vi "PRISM_RasterScan_BSC202.vi"() -> ()   [LabVIEW 2022 SP3]
uses:
  C:/Users/mnopl/Desktop/Software/mnOPSuite/PRISM/Thorlabs.MotionControl.Controls.dll
  Thorlabs.MotionControl.Controls.dll
  C:/Users/mnopl/Desktop/Software/mnOPSuite/PRISM/Thorlabs.MotionControl.Benchtop.StepperMotorCLI.dll
  Thorlabs.MotionControl.Benchtop.StepperMotorCLI.dll
  Control_PRISMRasterScan_ActivityLoop.ctl
  Control_PRISMRasterScan_ProtocolsLoop.ctl
  Control_LineScanCounterAE.ctl
  <vilib>/Analysis/baseanly.llb/Mean (DBL).vi
  C:/Users/mnopl/Desktop/Software/mnOPSuite/PRISM/Thorlabs.MotionControl.KCube.StepperMotorCLI.dll
  Thorlabs.MotionControl.KCube.StepperMotorCLI.dll
  <vilib>/Analysis/NI_AALBase.lvlib
panel:
  in  "Update origin":bool
  out "Protocol status":string="Ready for protocol!"
  in  "Protocols":T1(tab)
  in  "Target coordinate":T2={"X coord (mm)"=10.4027, "Y coord (mm)"=14.895, "Z coord (mm)"=19.058}
  in  "Move to target":bool
  out "Origin coordinate":T2={"X coord (mm)"=10.4027001953125, "Y coord (mm)"=14.895, "Z coord (mm)"=19.057761655908987}
  in  "Update target":bool
  in  "Move to origin":bool
  in  "Stored positions":T3(array[cluster])=[{"X coord (mm)"=10.4027, "Y coord (mm)"=14.895, "Z coord (mm)"=19.058}, {"X coord (mm)"=4.4859619140625, "Y coord (mm)"=8.22592529296875, "Z coord (mm)"=18.22813350697374}, {"X coord (mm)"=9.08337158203125, "Y coord (mm)"=16.38648681640625, "Z coord (mm)"=19.027052048324006}]
  in  "Stored position names":string[](array[string])=["SSO Center", "Gold", "Shane region"]
  in  "Move to\nstored position":bool[](array[boolean])=[FALSE, FALSE, FALSE]
  in  "Store target\nposition to":bool[](array[boolean])=[FALSE, FALSE, FALSE]
  in  "Do Linescan":bool
  in  "Linescan points\n(relative x,y, microns)":dbl[][](array[numeric])=[[1973.4850685095644, -1528.847563473508], [1962.5356538406427, -1517.3322023102946], [1951.5862391717208, -1505.8168411470815], [1940.636824502799, -1494.3014799838681], [1929.6874098338772, -1482.786118820655], [1918.7379951649555, -1471.2707576574417], [1907.7885804960335, -1459.7553964942285], [1896.8391658271119, -1448.2400353310152], [1885.88975115819, -1436.7246741678018], [1874.9403364892682, -1425.2093130045887], [1863.9909218203463, -1413.6939518413753], [1853.0415071514246, -1402.1785906781622], [1842.0920924825027, -1390.6632295149489], [1831.142677813581, -1379.1478683517357], [1820.193263144659, -1367.6325071885224], [1809.2438484757374, -1356.117146025309], [1798.2944338068155, -1344.6017848620959], [1787.3450191378938, -1333.0864236988825], [1776.395604468972, -1321.5710625356694], [1765.4461898000502, -1310.055701372456], [1754.4967751311283, -1298.540340209243], [1743.5473604622066, -1287.0249790460296], [1732.597945793285, -1275.5096178828162], [1721.648531124363, -1263.994256719603], [1710.699116455441, -1252.4788955563897], [1699.7497017865194, -1240.9635343931764], [1688.8002871175977, -1229.4481732299632], [1677.8508724486758, -1217.93281206675], [1666.901457779754, -1206.4174509035367], [1655.9520431108322, -1194.9020897403234], [1645.0026284419105, -1183.3867285771103], [1634.0532137729886, -1171.871367413897], [1623.1037991040669, -1160.3560062506835], [1612.154384435145, -1148.8406450874704], [1601.2049697662233, -1137.325283924257], [1590.2555550973013, -1125.809922761044], [1579.3061404283796, -1114.2945615978306], [1568.3567257594577, -1102.7792004346175], [1557.407311090536, -1091.263839271404], [1546.4578964216144, -1079.7484781081907], [1535.5084817526924, -1068.2331169449776], [1524.5590670837705, -1056.7177557817643], [1513.6096524148488, -1045.2023946185511], [1502.6602377459271, -1033.6870334553378], [1491.7108230770052, -1022.1716722921245], [1480.7614084080833, -1010.6563111289113], [1469.8119937391616, -999.140949965698], [1458.86257907024, -987.6255888024848], [1447.913164401318, -976.1102276392714], [1436.963749732396, -964.5948664760582], [1426.0143350634744, -953.079505312845], [1415.0649203945527, -941.5641441496317], [1404.1155057256308, -930.0487829864185], [1393.1660910567089, -918.5334218232052], [1382.2166763877872, -907.018060659992], [1371.2672617188655, -895.5026994967786], [1360.3178470499438, -883.9873383335654], [1349.3684323810219, -872.4719771703521], [1338.4190177121, -860.9566160071389], [1327.4696030431783, -849.4412548439257]]
  in  "Linescan Accumulations":i32=10 min=1
  out "Current point":i32
  in  "Halt linescan":bool
  out "Current\naccumulation":i32=10
  in  "Generate\n# points\n(cursors 1&2)":bool
  in  "# Points":i32=60 min=2 max=100
  out "X stepper reference":refnum<k24>
  out "Y stepper reference":refnum<k24>
  in  "BenchtopStepperControl Y":refnum<k24>(container)
  in  "BenchtopStepperControl X":refnum<k24>(container)
  in  "Save Image":bool
  in  "Path to save image":path=path "D:/Dropbox/Data/PRISM/2022.12.15 - SSO film undopded - test linescans/SSO(Overall)@(14.25microns,Mono,45degrees)_phase.txt"
  in  "Move to cursor 1":bool
  in  "Auto-level phase":bool
  in  "Acquire":bool=TRUE
  in  "Settle Time Y":u32=500
  in  "2nd sideband factor":dbl=1.0
  in  "Settle Time X":u32=50
  in  "Py":dbl=1.385597069551572 format="%_3f"
  in  "Px":dbl=-9.353762914113396 format="%_3f"
  in  "1st sideband offset":dbl
  in  "Phase offset":dbl=-4.26501095307295 format="%_3f"
  out "Phase":dbl[][](graph)
  in  "SerialNumber Z":string="26004283"
  in  "KCubeStepperControl Z":refnum<k24>(container)
  in  "Num Of Steps X":i32=350
  in  "Num Of Steps Y":i32=350
  out "Amplitude":dbl[][](graph)
  in  "Integration time (s)":dbl=0.05
  in  "?":bool
  in  "?":bool
  in  "Halt program":bool=TRUE
  in  "Step Size X (um)":sgl=15.0 format="%.8f"
  in  "SerialNumber X":string="70283584"
  in  "Step Size Y (um)":sgl=15.0 format="%.8f"
  in  "SerialNumber Y":string="70283584"
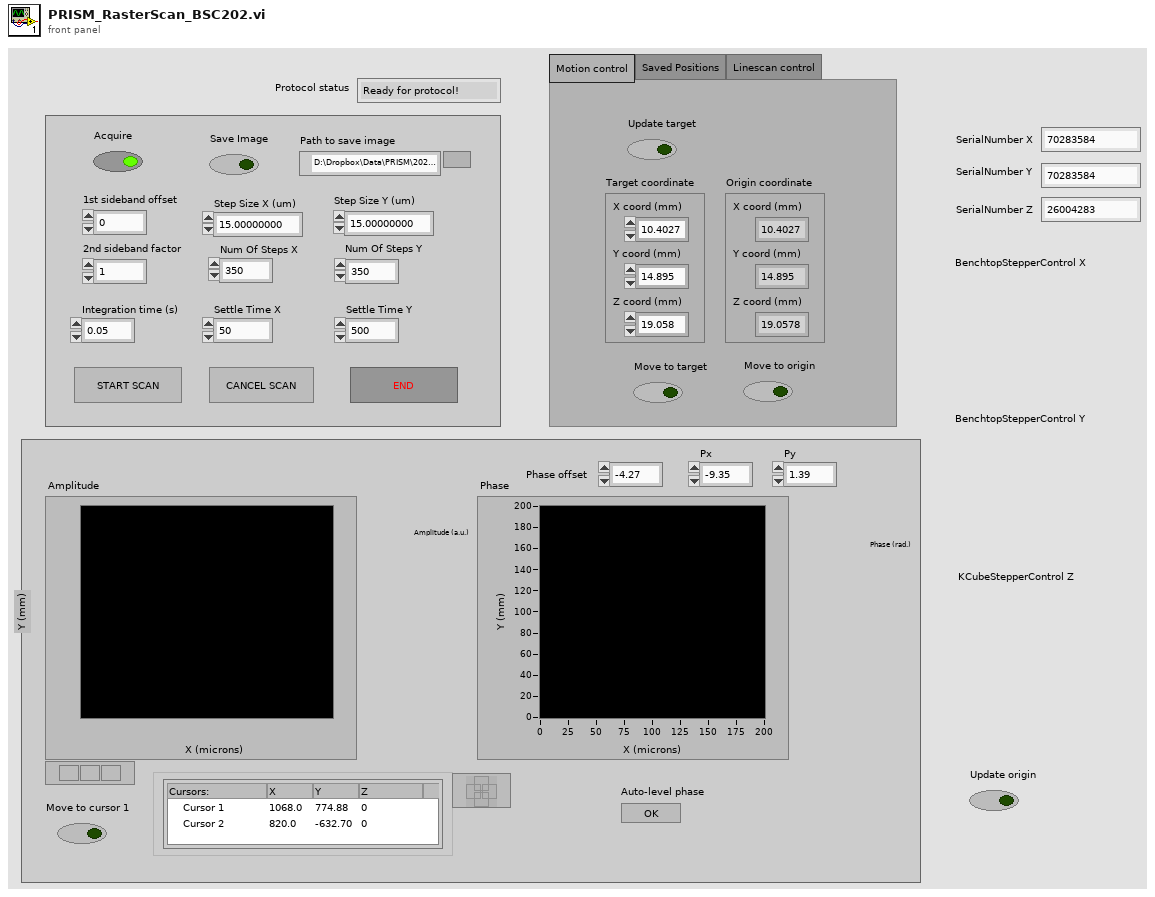
[diagram p1: front panel]
types:
  T1 = enum32{"Motion control", "Saved Positions", "Linescan control"}
  T2 = cluster{"X coord (mm)":dbl, "Y coord (mm)":dbl, "Z coord (mm)":dbl}
  T3 = cluster{"X coord (mm)":dbl, "Y coord (mm)":dbl, "Z coord (mm)":dbl}[]
  T4 = typedef "Control_PRISMRasterScan_ProtocolsLoop.ctl" = enum16{"Sit Idle", "Generate linescan points", "Initialize Linescan", "Update Linescan target", "Move linescan and wait", "Finalize linescan", "Move to stored position", "Store target position"}
  T5 = typedef "Control_PRISMRasterScan_ActivityLoop.ctl" = enum16{"Sit Idle", "Move to target", "Update origin or target position", "Move to origin"}
  T6 = typedef "Control_LineScanCounterAE.ctl" = enum16{"Initialize", "Activate", "Attach indicators", "Increment Point", "Query", "Do Finish Point", "Acknowledge line", "Deactivate"}
  T7 = typedef "LVCursorListTypeDef.ctl" = cluster{"Name":string, "Color":u32, "Style":u8, "Point Style":u8, "Name Visible":bool, "Allow Drag":bool, "Cursor Mode":u32, "Plot":i32, "Index":i32, "Position":cluster{"X":dbl, "Y":dbl}, "X Scale":u32, "Y Scale":u32, "Watch Plots":i32[], "Watch All Plots":bool, "Plot Area":i32, "Label Offset":cluster{"X":dbl, "Y":dbl}}[]
  T8 = cluster{"Name":string, "Color":u32, "Style":u8, "Point Style":u8, "Name Visible":bool, "Allow Drag":bool, "Cursor Mode":u32, "Plot":i32, "Index":i32, "Position":cluster{"X":dbl, "Y":dbl}, "X Scale":u32, "Y Scale":u32, "Watch Plots":i32[], "Watch All Plots":bool, "Plot Area":i32, "Label Offset":cluster{"X":dbl, "Y":dbl}}
  T9 = typedef "imagedata.ctl" = cluster{"image type":i32, "image depth":i32, "image":u8[], "mask":u8[], "colors":u32[], "Rectangle":cluster{"left":i16, "top":i16, "right":i16, "bottom":i16}}
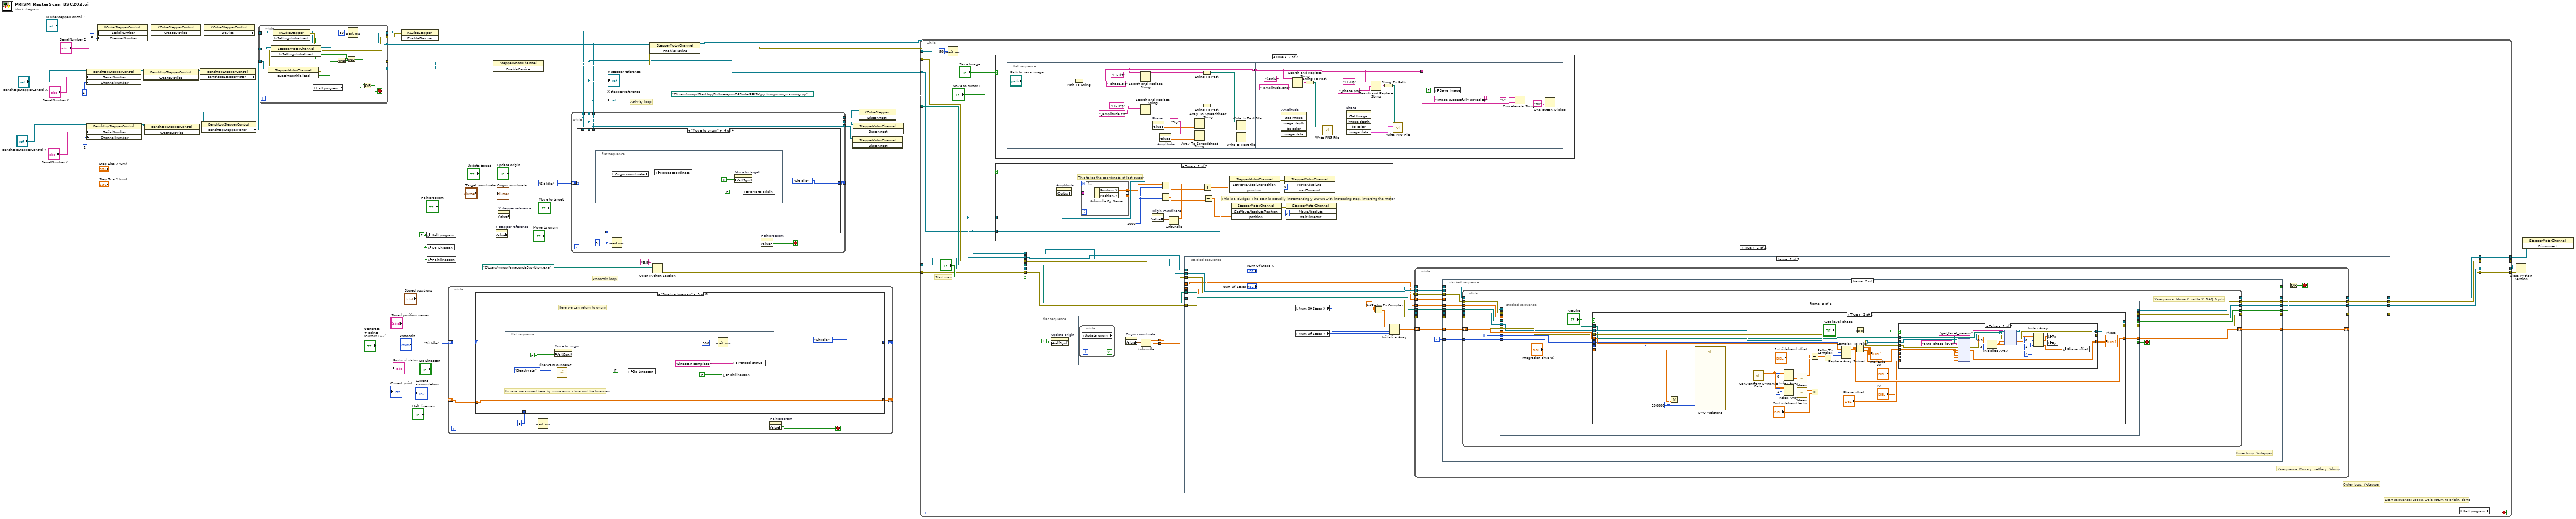
[diagram p0: block diagram]
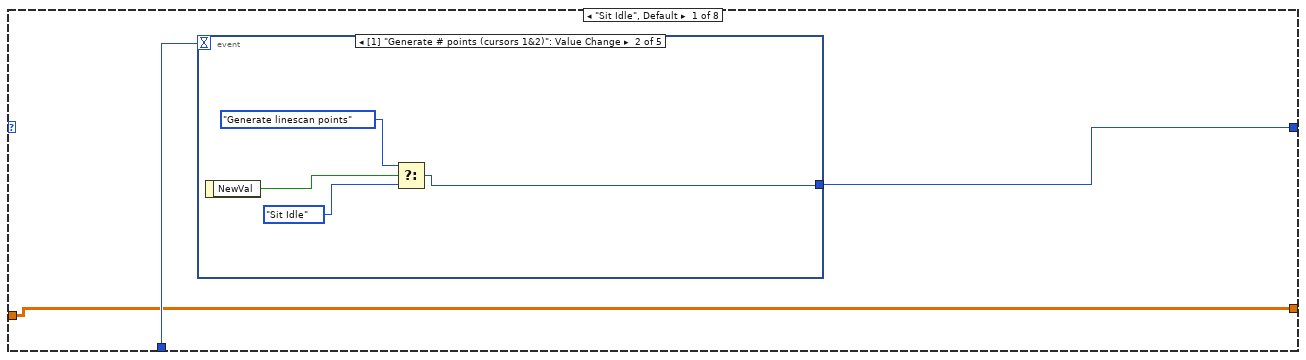
[diagram p2: hidden frame]
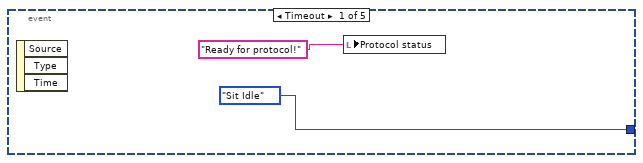
[diagram p3: hidden frame]
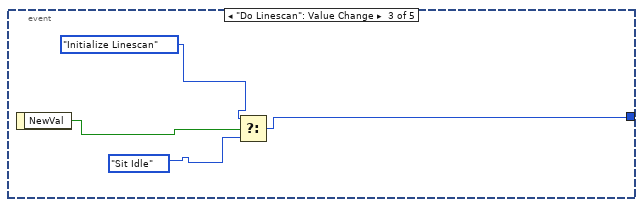
[diagram p4: hidden frame]
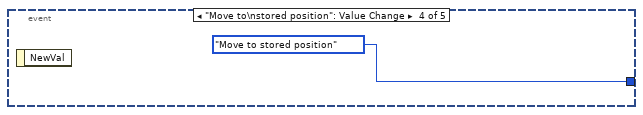
[diagram p5: hidden frame]
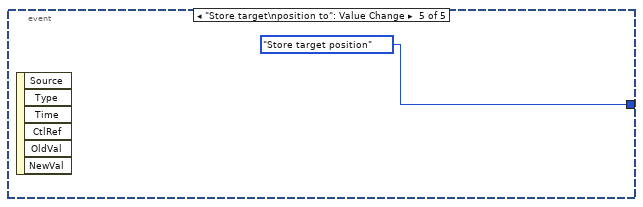
[diagram p6: hidden frame]
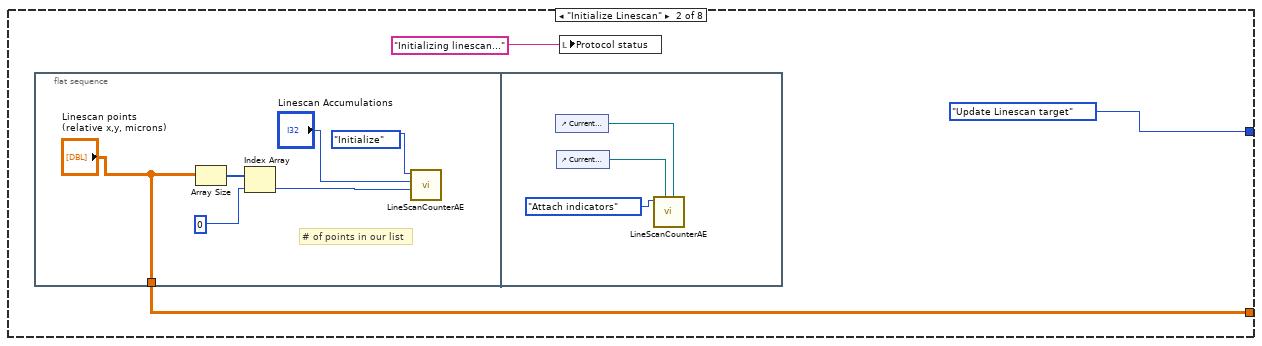
[diagram p7: hidden frame]
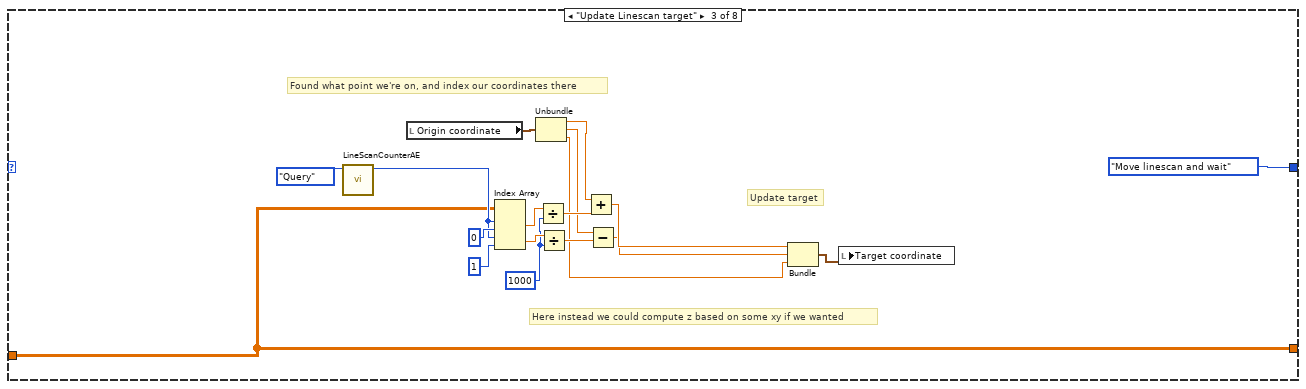
[diagram p8: hidden frame]
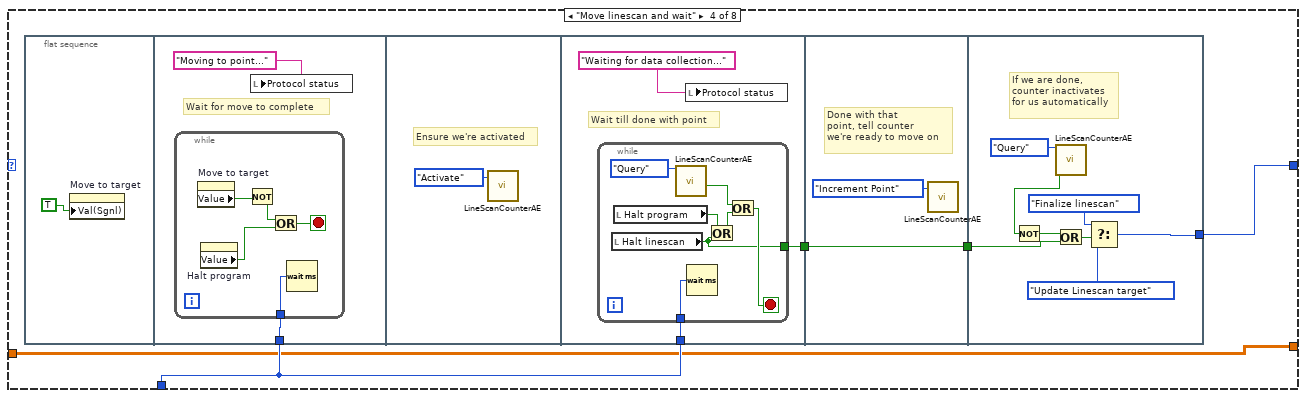
[diagram p9: hidden frame]
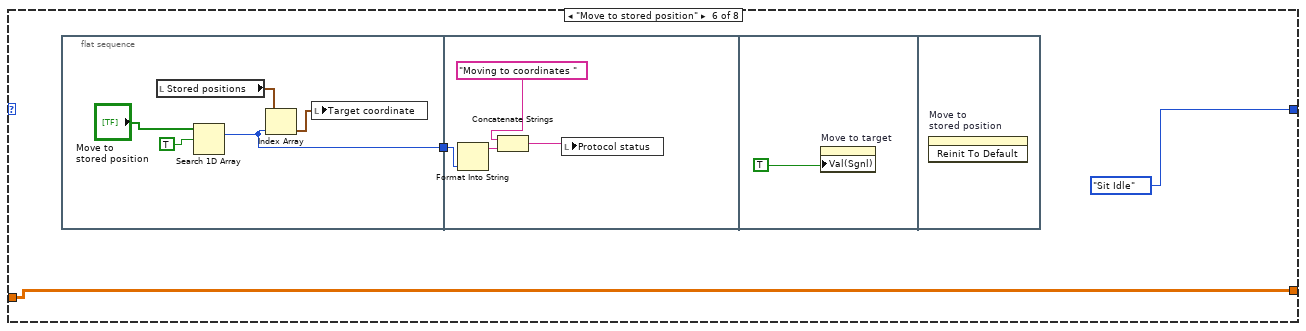
[diagram p10: hidden frame]
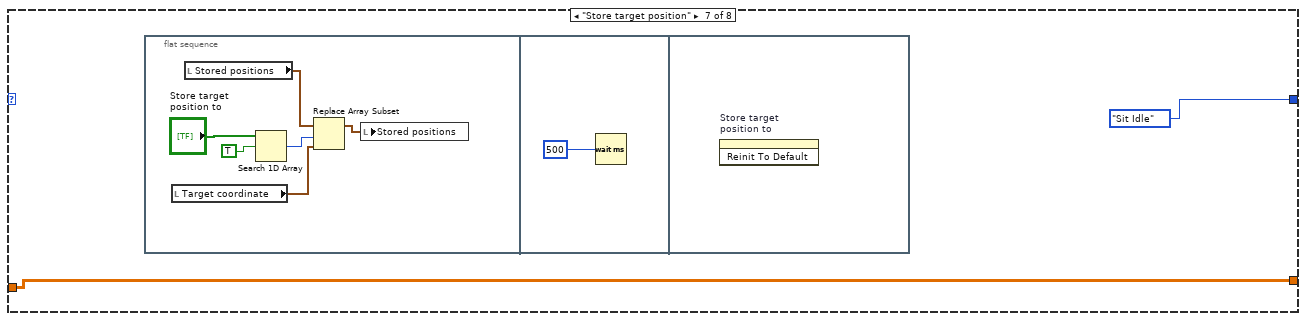
[diagram p11: hidden frame]
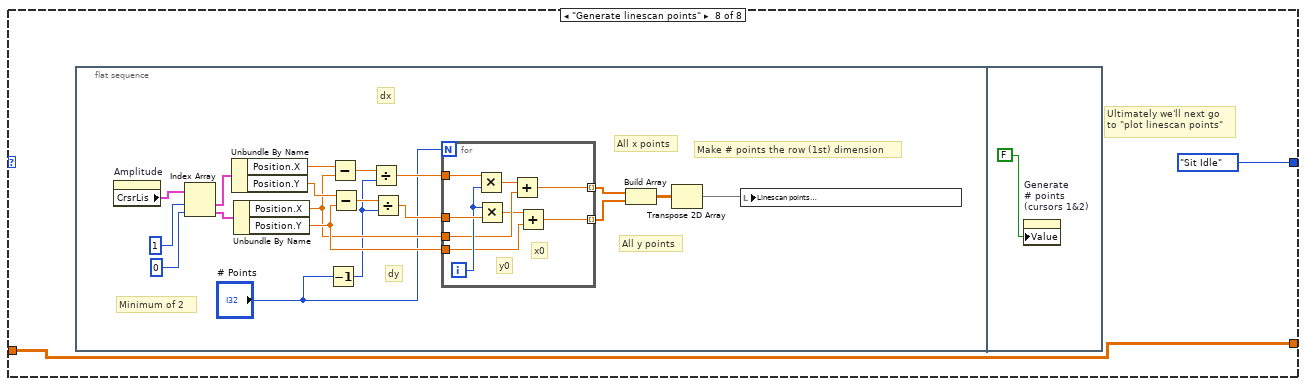
[diagram p12: hidden frame]
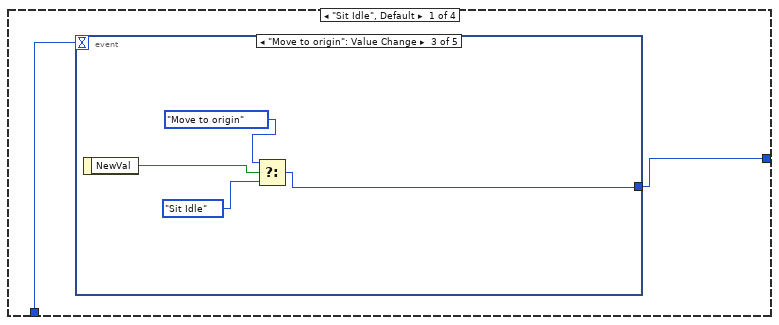
[diagram p13: hidden frame]
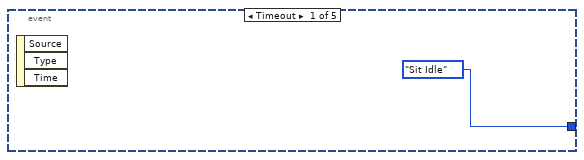
[diagram p14: hidden frame]
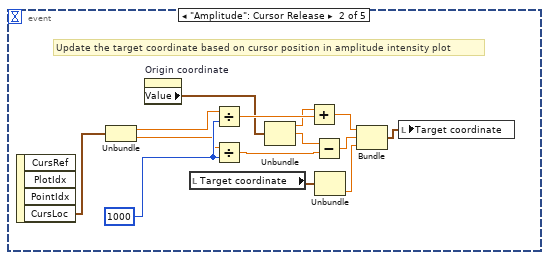
[diagram p15: hidden frame]
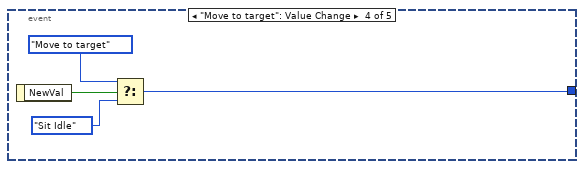
[diagram p16: hidden frame]
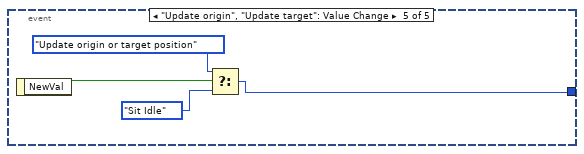
[diagram p17: hidden frame]
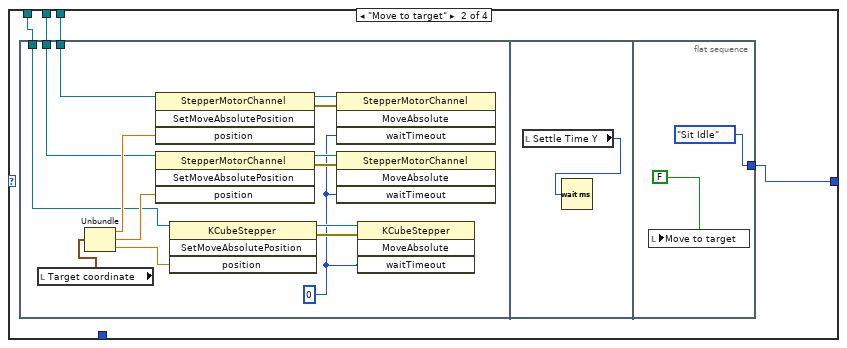
[diagram p18: hidden frame]
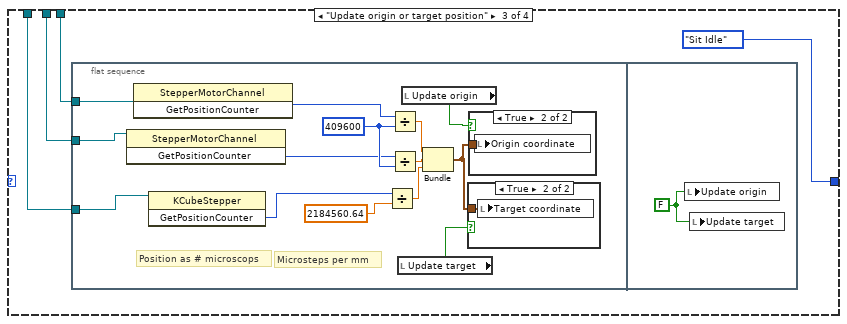
[diagram p19: hidden frame]
diagram:
  w7 = FALSE
  # "Protocols loop"
  # "Activity loop"
  n1 = property class="BenchtopStepperControl"(reference="BenchtopStepperControl X", "SerialNumber"="SerialNumber X", "ChannelNumber"=1) -> (reference out=w13:refnum<k24>)  [unwired: 1 in, 1 out]
  n2 = property class="BenchtopStepperControl"(reference="BenchtopStepperControl Y", "SerialNumber"="SerialNumber Y", "ChannelNumber"=2) -> (reference out=w12:refnum<k24>)  [unwired: 1 in, 1 out]
  n3 = property class="KCubeStepperControl"(reference="KCubeStepperControl Z", "SerialNumber"="SerialNumber Z", "ChannelNumber"=3) -> (reference out=w35:refnum<k24>)  [unwired: 1 in, 1 out]
  n4 = invoke class="BenchtopStepperControl" method="CreateDevice"(reference=w13) -> (reference out=w42:refnum<k24>)  [unwired: 2 in, 2 out]
  n5 = invoke class="BenchtopStepperControl" method="CreateDevice"(reference=w12) -> (reference out=w43:refnum<k24>)  [unwired: 2 in, 2 out]
  n6 = invoke class="KCubeStepperControl" method="CreateDevice"(reference=w35) -> (reference out=w34:refnum<k24>)  [unwired: 2 in, 2 out]
  n7 = property class="BenchtopStepperControl"(reference=w42) -> ("BenchtopStepperMotor"=w41:refnum<k24>)  [unwired: 1 in, 2 out]
  n8 = property class="BenchtopStepperControl"(reference=w43) -> ("BenchtopStepperMotor"=w27:refnum<k24>)  [unwired: 1 in, 2 out]
  n9 = property class="KCubeStepperControl"(reference=w34) -> ("Device"=w29:refnum<k24>)  [unwired: 1 in, 2 out]
  n10 = while {
    tunnel: w27 -> [w50]
    tunnel: w41 -> [w54]
    tunnel: [w52] -> w40
    tunnel: [w48] -> w39
    tunnel: [w53] -> w1
    tunnel: [w56] -> w31
    tunnel: [w57] -> w30
    tunnel: w29 -> [w58]
    stop <- w44 stop-if-true
    n11 = invoke class="StepperMotorChannel" method="IsSettingsInitialized"(reference=w50) -> (reference out=w48:refnum<k24>, error out=w49:errorcluster, "IsSettingsInitialized"=w47:bool)  [unwired: 2 in]
    n12 = invoke class="StepperMotorChannel" method="IsSettingsInitialized"(reference=w54, error in=w49) -> (reference out=w53:refnum<k24>, error out=w52:errorcluster, "IsSettingsInitialized"=w51:bool)  [unwired: 1 in]
    n13 = invoke class="KCubeStepper" method="IsSettingsInitialized"(reference=w58) -> (reference out=w56:refnum<k24>, error out=w57:errorcluster, "IsSettingsInitialized"=w55:bool)  [unwired: 2 in]
    n14 = local read "Halt program"() -> (w46:bool)
    n15 = And(x=w55, y=w47) -> (x .and. y?=w59:bool)
    n16 = And(x=w51, y=w59) -> (x .and. y?=w45:bool)
    n17 = Wait (ms)(milliseconds to wait=u32 50) -> ()  [unwired: 1 out]
    n18 = Or(x=w45, y=w46) -> (x .or. y?=w44:bool)
  }
  "X stepper reference" <- w1
  n19 = invoke class="KCubeStepper" method="EnableDevice"(reference=w31, error in=w30) -> (reference out=w5:refnum<k24>)  [unwired: 1 in, 2 out]
  n20 = local write "Halt program"(w7) -> ()
  n21 = local write "Do Linescan"(w7) -> ()
  n22 = local write "Halt linescan"(w7) -> ()
  n23 = while {
    shift-right: [w64] -> _
    shift-left: Control_PRISMRasterScan_ProtocolsLoop."Sit Idle" -> [w61]
    shift-right: [w63] -> _
    shift-left: _ -> [w62]
    stop <- w66 stop-if-true
    w65 = 5
    n24 = case shown="\"Finalize linescan\"" w61 {
      tunnel: w65 -> [w69 _ _ w116 _ _ _ _]
      tunnel: [w68 Control_PRISMRasterScan_ProtocolsLoop."Update Linescan target" Control_PRISMRasterScan_ProtocolsLoop."Move linescan and wait" w115 Control_PRISMRasterScan_ProtocolsLoop."Sit Idle" Control_PRISMRasterScan_ProtocolsLoop."Sit Idle" Control_PRISMRasterScan_ProtocolsLoop."Sit Idle" Control_PRISMRasterScan_ProtocolsLoop."Sit Idle"] -> w64
      tunnel: [w67 w83 w99 w112 w146 w155 w167 w176] -> w63
      tunnel: w62 -> [w67 _ w99 w112 w146 w155 w167 w176]
      frame "Sit Idle", Default {
        n25 = event shown="[1] \"Generate # points (cursors 1&2)\": Value Change" {
          selector: _ -> [_ _ _ _ _]
          dyn-events: _ -> [_ _ _ _ _]
          timeout: w69 -> [_ _ _ _ _]
          tunnel: [Control_PRISMRasterScan_ProtocolsLoop."Sit Idle" w72 w78 Control_PRISMRasterScan_ProtocolsLoop."Move to stored position" Control_PRISMRasterScan_ProtocolsLoop."Store target position"] -> w68
          event Timeout {
            n26 = event-data() -> ()  [unwired: 1 in, 3 out]
            n27 = local write "Protocol status"("Ready for protocol!") -> ()
          }
          event "Generate\n# points\n(cursors 1&2)": Value Change {
            n28 = event-data() -> ("NewVal"=w75:bool)  [unwired: 1 in]
            n29 = Select(t=Control_PRISMRasterScan_ProtocolsLoop."Generate linescan points", s=w75, f=Control_PRISMRasterScan_ProtocolsLoop."Sit Idle") -> (s? t:f=w72:T4)
          }
          event "Do Linescan": Value Change {
            n30 = event-data() -> ("NewVal"=w79:bool)  [unwired: 1 in]
            n31 = Select(t=Control_PRISMRasterScan_ProtocolsLoop."Initialize Linescan", s=w79, f=Control_PRISMRasterScan_ProtocolsLoop."Sit Idle") -> (s? t:f=w78:T4)
          }
          event "Move to\nstored position": Value Change {
            n32 = event-data() -> ()  [unwired: 1 in, 1 out]
          }
          event "Store target\nposition to": Value Change {
            n33 = event-data() -> ()  [unwired: 1 in, 6 out]
          }
        }
      }
      frame "Initialize Linescan" {
        n34 = flat-sequence {
          tunnel: ["Linescan points\n(relative x,y, microns)"] -> w83
          frame #0 {
            # "# of points in our list"
            n35 = Array Size(array="Linescan points\n(relative x,y, microns)") -> (size(s)=w90:i32[])
            n36 = Index Array(array=w90, index=0) -> (element=w89:i32)
            n37 = call "LineScanCounterAE.vi"("Number of points"=w89, "Accumulate to #"="Linescan Accumulations", "Task"=Control_LineScanCounterAE."Initialize") -> ()  [unwired: 2 in, 7 out]
          }
          frame #1 {
            n38 = control-ref of="Current\naccumulation"() -> (w92:refnum<vi>)
            n39 = control-ref of="Current point"() -> (w91:refnum<vi>)
            n40 = call "LineScanCounterAE.vi"("# Accumulated (reference)"=w92, "Current point index (reference)"=w91, "Task"=Control_LineScanCounterAE."Attach indicators") -> ()  [unwired: 2 in, 7 out]
          }
        }
        n41 = local write "Protocol status"("Initializing linescan...") -> ()
      }
      frame "Update Linescan target" {
        w102 = 1000
        # "Here instead we could compute z based on some xy if we wanted"
        # "Found what point we're on, and index our coordinates there"
        # "Update target"
        n42 = call "LineScanCounterAE.vi"("Task"=Control_LineScanCounterAE."Query" ("Enum")) -> ("Current point index"=w100:i32)  [unwired: 4 in, 6 out]
        n43 = local read "Origin coordinate"() -> (w97:T2)
        n44 = Index Array(array=w99, index (row) #1=w100, index (col) #1=0, index (row) #2=w100, index (col) #2=1) -> (element #1=w111:dbl, element #2=w110:dbl)
        n45 = Unbundle(w97) -> ("X coord (mm)"=w94:dbl, "Y coord (mm)"=w95:dbl, "Z coord (mm)"=w96:dbl)
        n46 = Divide(x=w111, y=w102) -> (x/y=w108:dbl)
        n47 = Divide(x=w110, y=w102) -> (x/y=w109:dbl)
        n48 = Add(x=w94, y=w108) -> (x+y=w107:dbl)
        n49 = Subtract(x=w95, y=w109) -> (x-y=w106:dbl)
        n50 = Bundle(w107, w106, "Z coord (mm)"=w96) -> (w105:cluster{dbl, dbl, "Z coord (mm)":dbl})  [unwired: 1 in]
        n51 = local write "Target coordinate"(w105) -> ()
      }
      frame "Move linescan and wait" {
        n52 = flat-sequence {
          tunnel: w116 -> [w119]
          tunnel: w116 -> [w128]
          tunnel: [w126] -> w113
          tunnel: [w136] -> w114
          tunnel: w113 -> [w136]
          tunnel: [w144] -> w115
          tunnel: w114 -> [w142]
          frame #0 {
            n53 = property on="Move to target" class="Bool (strict)"("Val(Sgnl)"=TRUE) -> ()  [unwired: 2 in, 2 out]
          }
          frame #1 {
            # "Wait for move to complete"
            n54 = while {
              tunnel: w119 -> [w120]
              stop <- w121 stop-if-true
              n55 = property on="Move to target" class="Bool (strict)"() -> ("Value"=w124:bool)  [unwired: 2 in, 2 out]
              n56 = property on="Halt program" class="Bool (strict)"() -> ("Value"=w122:bool)  [unwired: 2 in, 2 out]
              n57 = Not(x=w124) -> (.not. x?=w123:bool)
              n58 = Or(x=w123, y=w122) -> (x .or. y?=w121:bool)
              n59 = Wait (ms)(milliseconds to wait=w120) -> ()  [unwired: 1 out]
            }
            n60 = local write "Protocol status"("Moving to point...") -> ()
          }
          frame #2 {
            # "Ensure we're activated"
            n61 = call "LineScanCounterAE.vi"("Task"=Control_LineScanCounterAE."Activate") -> ()  [unwired: 4 in, 7 out]
          }
          frame #3 {
            # "Wait till done with point"
            n62 = while {
              tunnel: w128 -> [w134]
              tunnel: [w129] -> w126
              stop <- w132 stop-if-true
              n63 = local read "Halt linescan"() -> (w129:bool)
              n64 = local read "Halt program"() -> (w133:bool)
              n65 = call "LineScanCounterAE.vi"("Task"=Control_LineScanCounterAE."Query") -> ("Done with point"=w130:bool)  [unwired: 4 in, 6 out]
              n66 = Wait (ms)(milliseconds to wait=w134) -> ()  [unwired: 1 out]
              n67 = Or(x=w133, y=w129) -> (x .or. y?=w131:bool)
              n68 = Or(x=w130, y=w131) -> (x .or. y?=w132:bool)
            }
            n69 = local write "Protocol status"("Waiting for data collection...") -> ()
          }
          frame #4 {
            # "Done with that\npoint, tell counter\nwe're ready to move on"
            n70 = call "LineScanCounterAE.vi"("Task"=Control_LineScanCounterAE."Increment Point") -> ()  [unwired: 4 in, 7 out]
          }
          frame #5 {
            # "If we are done,\ncounter inactivates\nfor us automatically"
            n71 = call "LineScanCounterAE.vi"("Task"=Control_LineScanCounterAE."Query") -> ("Active"=w140:bool)  [unwired: 4 in, 6 out]
            n72 = Not(x=w140) -> (.not. x?=w141:bool)
            n73 = Or(x=w141, y=w142) -> (x .or. y?=w143:bool)
            n74 = Select(t=Control_PRISMRasterScan_ProtocolsLoop."Finalize linescan", s=w143, f=Control_PRISMRasterScan_ProtocolsLoop."Update Linescan target") -> (s? t:f=w144:T4)
          }
        }
      }
      frame "Finalize linescan" {
        # "In case we arrived here by some error, close out the linescan"
        # "Here we can return to origin"
        n75 = flat-sequence {
          frame #0 {
            n76 = property on="Move to origin" class="Bool (strict)"("Val(Sgnl)"=FALSE) -> ()  [unwired: 2 in, 2 out]
            n77 = call "LineScanCounterAE.vi"("Task"=Control_LineScanCounterAE."Deactivate" ("Enum")) -> ()  [unwired: 4 in, 7 out]
          }
          frame #1 {
            n78 = local write "Do Linescan"(FALSE) -> ()
          }
          frame #2 {
            n79 = Wait (ms)(milliseconds to wait=500) -> ()  [unwired: 1 out]
            n80 = local write "Halt linescan"(FALSE) -> ()
            n81 = local write "Protocol status"("Linescan complete!") -> ()
          }
        }
      }
      frame "Move to stored position" {
        n82 = flat-sequence {
          tunnel: [w158] -> w154
          tunnel: w154 -> [w164]
          frame #0 {
            n83 = local read "Stored positions"() -> (w157:T3)
            n84 = Search 1D Array(1D array="Move to\nstored position", element=TRUE) -> (index of element=w158:i32)  [unwired: 1 in]
            n85 = Index Array(array=w157, index=w158) -> (element=w159:T2)
            n86 = local write "Target coordinate"(w159) -> ()
          }
          frame #1 {
            n87 = Format Into String(w164) -> (resulting string=w163:string)  [unwired: 3 in, 1 out]
            n88 = Concatenate Strings("Moving to coordinates ", w163) -> (w162:string)
            n89 = local write "Protocol status"(w162) -> ()
          }
          frame #2 {
            n90 = property on="Move to target" class="Bool (strict)"("Val(Sgnl)"=TRUE) -> ()  [unwired: 2 in, 2 out]
          }
          frame #3 {
            n91 = invoke on="Move to\nstored position" class="Arr (strict)" method="Reinit To Default"() -> ()  [unwired: 3 in, 3 out]
          }
        }
      }
      frame "Store target position" {
        n92 = flat-sequence {
          frame #0 {
            n93 = local read "Target coordinate"() -> (w170:T2)
            n94 = local read "Stored positions"() -> (w169:T3)
            n95 = Search 1D Array(1D array="Store target\nposition to", element=TRUE) -> (index of element=w172:i32)  [unwired: 1 in]
            n96 = Replace Array Subset(array=w169, new element=w170, index=w172) -> (w171:T3)
            n97 = local write "Stored positions"(w171) -> ()
          }
          frame #1 {
            n98 = Wait (ms)(milliseconds to wait=500) -> ()  [unwired: 1 out]
          }
          frame #2 {
            n99 = invoke on="Store target\nposition to" class="Arr (strict)" method="Reinit To Default"() -> ()  [unwired: 3 in, 3 out]
          }
        }
      }
      frame "Generate linescan points" {
        # "Ultimately we'll next go \nto \"plot linescan points\""
        n100 = flat-sequence {
          frame #0 {
            # "Minimum of 2"
            # "dy"
            # "dx"
            # "Make # points the row (1st) dimension"
            # "All y points"
            # "All x points"
            n101 = property on="Amplitude" class="IntGraph (strict)"() -> ("CrsrLis"=w196:T7)  [unwired: 2 in, 2 out]
            n102 = Index Array(array=w196, index #1=1, index #2=0) -> (element #1=w192:T8, element #2=w193:T8)
            n103 = Unbundle By Name(w192) -> ("Position.X"=w191:dbl, "Position.Y"=w190:dbl)
            n104 = Unbundle By Name(w193) -> ("Position.X"=w186:dbl, "Position.Y"=w187:dbl)
            n105 = Decrement(x="# Points") -> (x-1=w178:i32)
            n106 = Subtract(x=w191, y=w186) -> (x-y=w189:dbl)
            n107 = Subtract(x=w190, y=w187) -> (x-y=w188:dbl)
            n108 = Divide(x=w189, y=w178) -> (x/y=w184:dbl)
            n109 = Divide(x=w188, y=w178) -> (x/y=w185:dbl)
            n110 = for {
              N: "# Points" -> [_]
              tunnel: w187 -> [w200]
              tunnel: w186 -> [w201]
              tunnel: w185 -> [w205]
              tunnel: w184 -> [w203]
              tunnel: [w198] -> w183 mode=indexing
              tunnel: [w197] -> w182 mode=indexing
              i -> [w204]
              # "x0"
              # "y0"
              n111 = Multiply(x=w203, y=w204) -> (x*y=w202:dbl)
              n112 = Multiply(x=w204, y=w205) -> (x*y=w199:dbl)
              n113 = Add(x=w202, y=w201) -> (x+y=w198:dbl)
              n114 = Add(x=w199, y=w200) -> (x+y=w197:dbl)
            }
            n115 = Build Array(w183, w182) -> (w180:dbl[][])
            n116 = Transpose 2D Array(2D array=w180) -> (transposed array=w181:dbl[][])
            n117 = local write "Linescan points\n(relative x,y, microns)"(w181) -> ()
          }
          frame #1 {
            n118 = property on="Generate\n# points\n(cursors 1&2)" class="Bool (strict)"("Value"=FALSE) -> ()  [unwired: 2 in, 2 out]
          }
        }
      }
    }
    n119 = Wait (ms)(milliseconds to wait=w65) -> ()  [unwired: 1 out]
    n120 = property on="Halt program" class="Bool (strict)"() -> ("Value"=w66:bool)  [unwired: 2 in, 2 out]
  }
  n121 = invoke class="StepperMotorChannel" method="EnableDevice"(reference=w39, error in=w40) -> (reference out=w8:refnum<k24>, error out=w38:errorcluster)  [unwired: 1 in, 1 out]
  "Y stepper reference" <- w8
  n122 = property on="Y stepper reference" class="Ref (strict)" props=["Value"]() -> ()  [unwired: 2 in, 3 out]
  n123 = property on="X stepper reference" class="Ref (strict)" props=["Value"]() -> ()  [unwired: 2 in, 3 out]
  n124 = while {
    shift-right: [w212] -> _
    shift-left: Control_PRISMRasterScan_ActivityLoop."Sit Idle" -> [w213]
    tunnel: w8 -> [w208]
    tunnel: w1 -> [w207]
    tunnel: w5 -> [w209]
    tunnel: [w209] -> w4
    tunnel: [w208] -> w3
    tunnel: [w207] -> w2
    stop <- w211 stop-if-true
    w210 = 5
    n125 = case shown="\"Move to origin\"" w213 {
      tunnel: [w215 w246 Control_PRISMRasterScan_ActivityLoop."Sit Idle" Control_PRISMRasterScan_ActivityLoop."Sit Idle"] -> w212
      tunnel: w210 -> [w214 _ _ _]
      tunnel: w208 -> [_ w245 w266 _]
      tunnel: w207 -> [_ w244 w265 _]
      tunnel: w209 -> [_ w243 w267 _]
      frame "Sit Idle", Default {
        n126 = event shown="[2] \"Move to origin\": Value Change" {
          selector: _ -> [_ _ _ _ _]
          dyn-events: _ -> [_ _ _ _ _]
          timeout: w214 -> [_ _ _ _ _]
          tunnel: [Control_PRISMRasterScan_ActivityLoop."Sit Idle" _ w231 w235 w239] -> w215
          event Timeout {
            n127 = event-data() -> ()  [unwired: 1 in, 3 out]
          }
          event "Amplitude": Cursor Release {
            w224 = 1000
            # "Update the target coordinate based on cursor position in amplitude intensity plot"
            n128 = event-data() -> ("CursLoc"=w230:cluster{"X":dbl, "Y":dbl})  [unwired: 1 in, 3 out]
            n129 = Unbundle(w230) -> ("X"=w223:dbl, "Y"=w222:dbl)
            n130 = property on="Origin coordinate" class="Clust (strict)"() -> ("Value"=w219:T2)  [unwired: 2 in, 2 out]
            n131 = local read "Target coordinate"() -> (w221:T2)
            n132 = Divide(x=w223, y=w224) -> (x/y=w229:dbl)
            n133 = Divide(x=w222, y=w224) -> (x/y=w228:dbl)
            n134 = Unbundle(w219) -> ("X coord (mm)"=w218:dbl, "Y coord (mm)"=w217:dbl)  [unwired: 1 out]
            n135 = Add(x=w218, y=w229) -> (x+y=w226:dbl)
            n136 = Subtract(x=w217, y=w228) -> (x-y=w227:dbl)
            n137 = Unbundle(w221) -> ("Z coord (mm)"=w220:dbl)  [unwired: 2 out]
            n138 = Bundle(w226, w227, "Z coord (mm)"=w220) -> (w225:cluster{dbl, dbl, "Z coord (mm)":dbl})  [unwired: 1 in]
            n139 = local write "Target coordinate"(w225) -> ()
          }
          event "Move to origin": Value Change {
            n140 = event-data() -> ("NewVal"=w234:bool)  [unwired: 1 in]
            n141 = Select(t=Control_PRISMRasterScan_ActivityLoop."Move to origin", s=w234, f=Control_PRISMRasterScan_ActivityLoop."Sit Idle") -> (s? t:f=w231:T5)
          }
          event "Move to target": Value Change {
            n142 = event-data() -> ("NewVal"=w238:bool)  [unwired: 1 in]
            n143 = Select(t=Control_PRISMRasterScan_ActivityLoop."Move to target", s=w238, f=Control_PRISMRasterScan_ActivityLoop."Sit Idle") -> (s? t:f=w235:T5)
          }
          event "Update origin", "Update target": Value Change {
            n144 = event-data() -> ("NewVal"=w242:bool)  [unwired: 1 in]
            n145 = Select(t=Control_PRISMRasterScan_ActivityLoop."Update origin or target position", s=w242, f=Control_PRISMRasterScan_ActivityLoop."Sit Idle") -> (s? t:f=w239:T5)
          }
        }
      }
      frame "Move to target" {
        n146 = flat-sequence {
          tunnel: w245 -> [w254]
          tunnel: w244 -> [w253]
          tunnel: w243 -> [w250]
          tunnel: [Control_PRISMRasterScan_ActivityLoop."Sit Idle"] -> w246
          frame #0 {
            w247 = 0
            n147 = local read "Target coordinate"() -> (w252:T2)
            n148 = Unbundle(w252) -> ("X coord (mm)"=w257:dbl, "Y coord (mm)"=w256:dbl, "Z coord (mm)"=w251:dbl)
            n149 = invoke class="StepperMotorChannel" method="SetMoveAbsolutePosition"(reference=w253, "position"=w257) -> (reference out=w255:refnum<k24>, error out=w258:errorcluster)  [unwired: 2 in, 2 out]
            n150 = invoke class="StepperMotorChannel" method="SetMoveAbsolutePosition"(reference=w254, "position"=w256) -> (reference out=w260:refnum<k24>, error out=w259:errorcluster)  [unwired: 2 in, 2 out]
            n151 = invoke class="KCubeStepper" method="SetMoveAbsolutePosition"(reference=w250, "position"=w251) -> (reference out=w249:refnum<k24>, error out=w248:errorcluster)  [unwired: 2 in, 2 out]
            n152 = invoke class="StepperMotorChannel" method="MoveAbsolute"(reference=w255, error in=w258, "waitTimeout"=w247) -> ()  [unwired: 1 in, 4 out]
            n153 = invoke class="StepperMotorChannel" method="MoveAbsolute"(reference=w260, error in=w259, "waitTimeout"=w247) -> ()  [unwired: 1 in, 4 out]
            n154 = invoke class="KCubeStepper" method="MoveAbsolute"(reference=w249, error in=w248, "waitTimeout"=w247) -> ()  [unwired: 1 in, 4 out]
          }
          frame #1 {
            n155 = local read "Settle Time Y"() -> (w261:u32)
            n156 = Wait (ms)(milliseconds to wait=w261) -> ()  [unwired: 1 out]
          }
          frame #2 {
            n157 = local write "Move to target"(FALSE) -> ()
          }
        }
      }
      frame "Update origin or target position" {
        n158 = flat-sequence {
          tunnel: w267 -> [w272]
          tunnel: w266 -> [w273]
          tunnel: w265 -> [w274]
          frame #0 {
            w281 = 409600
            # "Position as # microscops"
            # "Microsteps per mm"
            n159 = invoke class="StepperMotorChannel" method="GetPositionCounter"(reference=w273) -> ("GetPositionCounter"=w279:i32)  [unwired: 2 in, 2 out]
            n160 = invoke class="StepperMotorChannel" method="GetPositionCounter"(reference=w274) -> ("GetPositionCounter"=w280:i32)  [unwired: 2 in, 2 out]
            n161 = invoke class="KCubeStepper" method="GetPositionCounter"(reference=w272) -> ("GetPositionCounter"=w275:i32)  [unwired: 2 in, 2 out]
            n162 = Divide(x=w275, y=2184560.64) -> (x/y=w276:dbl)
            n163 = Divide(x=w280, y=w281) -> (x/y=w278:dbl)
            n164 = Divide(x=w279, y=w281) -> (x/y=w277:dbl)
            n165 = local read "Update target"() -> (w269:bool)
            n166 = local read "Update origin"() -> (w270:bool)
            n167 = Bundle(w278, w277, w276) -> (w268:cluster{dbl, dbl, dbl})  [unwired: 1 in]
            n168 = case shown="True" w269 {
              tunnel: w268 -> [_ w282]
              frame False {
              }
              frame True {
                n169 = local write "Target coordinate"(w282) -> ()
              }
            }
            n170 = case shown="True" w270 {
              tunnel: w268 -> [_ w283]
              frame False {
              }
              frame True {
                n171 = local write "Origin coordinate"(w283) -> ()
              }
            }
          }
          frame #1 {
            w284 = FALSE
            n172 = local write "Update origin"(w284) -> ()
            n173 = local write "Update target"(w284) -> ()
          }
        }
      }
      frame "Move to origin" {
        n174 = flat-sequence {
          frame #0 {
            n175 = local read "Origin coordinate"() -> (w286:T2)
            n176 = local write "Target coordinate"(w286) -> ()
          }
          frame #1 {
            n177 = property on="Move to target" class="Bool (strict)"("Val(Sgnl)"=TRUE) -> ()  [unwired: 2 in, 2 out]
            n178 = local write "Move to origin"(FALSE) -> ()
          }
        }
      }
    }
    n179 = Wait (ms)(milliseconds to wait=w210) -> ()  [unwired: 1 out]
    n180 = property on="Halt program" class="Bool (strict)"() -> ("Value"=w211:bool)  [unwired: 2 in, 2 out]
  }
  n181 = invoke class="StepperMotorChannel" method="EnableDevice"(reference=w1, error in=w38) -> (reference out=w37:refnum<k24>, error out=w28:errorcluster)  [unwired: 1 in, 1 out]
  n182 = Open Python Session(python version="3.9", python path=path "C:/Users/mnopl/anaconda3/python.exe") -> (session out=w24:refnum<k35>, error out=w22:errorcluster)  [unwired: 1 in]
  n183 = invoke class="StepperMotorChannel" method="Disconnect"(reference=w2) -> ()  [unwired: 2 in, 3 out]
  n184 = invoke class="StepperMotorChannel" method="Disconnect"(reference=w3) -> ()  [unwired: 2 in, 3 out]
  n185 = invoke class="KCubeStepper" method="Disconnect"(reference=w4) -> ()  [unwired: 2 in, 3 out]
  n186 = while {
    tunnel: w8 -> [w291]
    tunnel: w37 -> [w292]
    tunnel: w28 -> [w301]
    tunnel: w24 -> [w300]
    tunnel: path "C:/Users/mnopl/Desktop/Software/mnOPSuite/PRISM/python/prism_scanning.py" -> [w299]
    tunnel: w22 -> [w298]
    tunnel: [w297] -> w21
    tunnel: [w296] -> w20
    tunnel: [w295] -> w19
    tunnel: [w294] -> w18
    stop <- w289 stop-if-true
    # "Start scan"
    n187 = Wait (ms)(milliseconds to wait=50) -> ()  [unwired: 1 out]
    n188 = case shown="True" "Save Image" {
      frame False {
      }
      frame True {
        n189 = flat-sequence {
          tunnel: [w306] -> w305
          tunnel: w305 -> [w321]
          tunnel: [w321] -> w304
          tunnel: w304 -> [w334]
          frame #0 {
            w314 = "%g"
            n190 = Path To String(path="Path to save image") -> (string=w306:string)
            n191 = Search and Replace String(input string=w306, search string="(.txt)$", replace string="_phase.txt") -> (result string=w319:string)  [unwired: 5 in, 3 out]
            n192 = Search and Replace String(input string=w306, search string="(.txt)*$", replace string="_amplitude.txt") -> (result string=w307:string)  [unwired: 5 in, 3 out]
            n193 = property on="Phase" class="IntGraph (strict)"() -> ("Value"=w309:dbl[][])  [unwired: 2 in, 2 out]
            n194 = property on="Amplitude" class="IntGraph (strict)"() -> ("Value"=w308:dbl[][])  [unwired: 2 in, 2 out]
            n195 = Array To Spreadsheet String(array=w309, 3:w314) -> (spreadsheet string=w320:string)  [unwired: 1 in]
            n196 = Array To Spreadsheet String(array=w308, 3:w314) -> (spreadsheet string=w315:string)  [unwired: 1 in]
            n197 = String To Path(string=w319) -> (path=w318:path)
            n198 = String To Path(string=w307) -> (path=w317:path)
            n199 = Write to Text File(file (use dialog)=w318, text=w320) -> ()  [unwired: 2 in, 3 out]
            n200 = Write to Text File(file (use dialog)=w317, text=w315) -> ()  [unwired: 2 in, 3 out]
          }
          frame #1 {
            n201 = invoke on="Amplitude" class="IntGraph (strict)" method="Get Image"() -> ("image data"=w327:T9)  [unwired: 6 in, 5 out]
            n202 = Search and Replace String(input string=w321, search string="(.txt)$", replace string="_amplitude.png") -> (result string=w329:string)  [unwired: 5 in, 3 out]
            n203 = String To Path(string=w329) -> (path=w328:path)
            n204 = call <vilib>:"Write PNG File.vi"("image data"=w327, "path to PNG file"=w328) -> ()  [unwired: 8 in, 2 out]
            n205 = invoke on="Phase" class="IntGraph (strict)" method="Get Image"() -> ("image data"=w323:T9)  [unwired: 6 in, 5 out]
            n206 = Search and Replace String(input string=w321, search string="(.txt)$", replace string="_phase.png") -> (result string=w324:string)  [unwired: 5 in, 3 out]
            n207 = String To Path(string=w324) -> (path=w322:path)
            n208 = call <vilib>:"Write PNG File.vi"("image data"=w323, "path to PNG file"=w322) -> ()  [unwired: 8 in, 2 out]
          }
          frame #2 {
            n209 = local write "Save Image"(FALSE) -> ()
            n210 = Concatenate Strings("Image successfully saved to:" ("message"), "\r", w334) -> (w335:string)
            n211 = One Button Dialog(message=w335, button name ("OK")="OK") -> ()  [unwired: 1 out]
          }
        }
      }
    }
    n212 = case shown="True" "Move to cursor 1" {
      tunnel: w292 -> [_ w351]
      tunnel: w291 -> [_ w347]
      frame False {
      }
      frame True {
        w345 = 1000
        # "This is a cludge:  The scan is actually incrementing y DOWN with increasing step, inverting the motor"
        # "This takes the coordinate of last cursor"
        n213 = property on="Amplitude" class="IntGraph (strict)"() -> ("CrsrLis"=w356:T7)  [unwired: 2 in, 2 out]
        n214 = for {
          tunnel: w356 -> [w359] mode=indexing
          tunnel: [w358] -> w344
          tunnel: [w357] -> w346
          n215 = Unbundle By Name(w359) -> ("Position.X"=w358:dbl, "Position.Y"=w357:dbl)
        }
        n216 = property on="Origin coordinate" class="Clust (strict)"() -> ("Value"=w340:T2)  [unwired: 2 in, 2 out]
        n217 = Divide(x=w344, y=w345) -> (x/y=w343:dbl)
        n218 = Divide(x=w346, y=w345) -> (x/y=w341:dbl)
        n219 = Unbundle(w340) -> ("X coord (mm)"=w339:dbl, "Y coord (mm)"=w338:dbl)  [unwired: 1 out]
        n220 = Add(x=w339, y=w343) -> (x+y=w352:dbl)
        n221 = Subtract(x=w338, y=w341) -> (x-y=w342:dbl)
        n222 = invoke class="StepperMotorChannel" method="SetMoveAbsolutePosition"(reference=w351, "position"=w352) -> (reference out=w355:refnum<k24>, error out=w354:errorcluster)  [unwired: 2 in, 2 out]
        n223 = invoke class="StepperMotorChannel" method="SetMoveAbsolutePosition"(reference=w347, "position"=w342) -> (reference out=w350:refnum<k24>, error out=w349:errorcluster)  [unwired: 2 in, 2 out]
        n224 = invoke class="StepperMotorChannel" method="MoveAbsolute"(reference=w355, error in=w354, "waitTimeout"=0) -> ()  [unwired: 1 in, 4 out]
        n225 = invoke class="StepperMotorChannel" method="MoveAbsolute"(reference=w350, error in=w349, "waitTimeout"=0) -> ()  [unwired: 1 in, 4 out]
      }
    }
    n226 = case shown="True" "?" {
      tunnel: w292 -> [w361 w368]
      tunnel: w291 -> [_ w367]
      tunnel: w301 -> [w360 w366]
      tunnel: w300 -> [w363 w375]
      tunnel: w299 -> [_ w374]
      tunnel: w298 -> [w362 w373]
      tunnel: [w363 w372] -> w297
      tunnel: [w362 w371] -> w296
      tunnel: [w361 w370] -> w295
      tunnel: [w360 w369] -> w294
      frame False {
      }
      frame True {
        # "Scan sequence: Loops, wait, return to origin, done"
        n227 = flat-sequence {
          tunnel: [w379] -> w365
          tunnel: [w378] -> w364
          frame #0 {
            n228 = property on="Update origin" class="Bool (strict)"("Val(Sgnl)"=TRUE) -> ()  [unwired: 2 in, 2 out]
          }
          frame #1 {
            n229 = while {
              stop <- w377 continue-if-true
              n230 = local read "Update origin"() -> (w377:bool)
            }
          }
          frame #2 {
            n231 = property on="Origin coordinate" class="Clust (strict)"() -> ("Value"=w380:T2)  [unwired: 2 in, 2 out]
            n232 = Unbundle(w380) -> ("X coord (mm)"=w379:dbl, "Y coord (mm)"=w378:dbl)  [unwired: 1 out]
          }
        }
        n233 = stacked-sequence {
          tunnel: w367 -> [_ w395 _ w590 _]
          tunnel: w364 -> [_ w392 _ w591 _]
          tunnel: w368 -> [_ w396 _ w589 _]
          tunnel: w366 -> [_ w397 _ _ _]
          tunnel: w365 -> [_ w391 _ w592 _]
          tunnel: w375 -> [_ w402 _ _ _]
          tunnel: w374 -> [_ w401 _ _ _]
          tunnel: w373 -> [_ w400 _ _ _]
          tunnel: [_ w399 _ _ _] -> w372
          tunnel: [_ w398 _ _ _] -> w371
          tunnel: [_ w394 _ _ _] -> w370
          tunnel: [_ w393 _ _ _] -> w369
          frame #0 {
            n234 = local read "Num Of Steps Y"() -> (w386:i32)
            n235 = local read "Num Of Steps X"() -> (w389:i32)
            n236 = local read "Step Size Y (um)"() -> (w382:sgl)
            n237 = local read "Step Size X (um)"() -> (w384:sgl)
            n238 = Divide(x=w386, y=-2) -> (x/y=w387:dbl)
            n239 = Divide(x=w389, y=-2) -> (x/y=w390:dbl)
            n240 = property on="Amplitude" class="IntGraph (strict)"("YScale.Multiplier"=w382) -> ()  [unwired: 2 in, 2 out]
            n241 = property on="Amplitude" class="IntGraph (strict)"("XScale.Multiplier"=w384) -> ()  [unwired: 2 in, 2 out]
            n242 = Multiply(x=w382, y=w387) -> (x*y=w381:dbl)
            n243 = Multiply(x=w384, y=w390) -> (x*y=w383:dbl)
            n244 = property on="Amplitude" class="IntGraph (strict)"("YScale.Offset"=w381) -> ()  [unwired: 2 in, 2 out]
            n245 = property on="Amplitude" class="IntGraph (strict)"("XScale.Offset"=w383) -> ()  [unwired: 2 in, 2 out]
          }
          frame #1 {
            w404 = 0.0
            # "Outer loop: Y-stepper"
            n246 = local read "Num Of Steps X"() -> (w406:i32)
            n247 = local read "Num Of Steps Y"() -> (w407:i32)
            n248 = Re/Im To Complex(1:w404, 2:w404) -> (0:w403:cdb)
            n249 = Initialize Array(w403, w406, w407) -> (w405:cdb[][])
            n250 = while {
              shift-right: [w422] -> _
              shift-left: w405 -> [w423]
              tunnel: [w421] -> w394
              tunnel: w402 -> [w414]
              tunnel: w401 -> [w409]
              tunnel: w400 -> [w420]
              tunnel: [w419] -> w399
              tunnel: [w418] -> w398
              tunnel: w397 -> [w416]
              tunnel: w396 -> [w413]
              tunnel: w395 -> [w412]
              tunnel: w392 -> [w411]
              tunnel: w391 -> [w410]
              tunnel: [w408] -> w393
              i -> [w415]
              stop <- w424 stop-if-true
              # "Y-sequence: Move y, settle y, X-loop"
              n251 = stacked-sequence {
                tunnel: w423 -> [_ w451]
                tunnel: w420 -> [_ w450]
                tunnel: [_ w458] -> w425
                tunnel: [_ w457] -> w422
                tunnel: [_ w456] -> w421
                tunnel: [_ w455] -> w419
                tunnel: [_ w454] -> w418
                tunnel: [w435 _] -> w417
                tunnel: w416 -> [w431 w453]
                tunnel: w415 -> [w426 w452]
                tunnel: w414 -> [_ w449]
                tunnel: w413 -> [_ w448]
                tunnel: w412 -> [w432 _]
                tunnel: w411 -> [w430 _]
                tunnel: w410 -> [_ w447]
                tunnel: w409 -> [_ w446]
                tunnel: [_ w445] -> w408
                frame #0 {
                  n252 = local read "Step Size Y (um)"() -> (w434:sgl)
                  n253 = local read "Num Of Steps Y"() -> (w440:i32)
                  n254 = Equal?(x=w426, y=w440) -> (x = y?=w438:bool)
                  n255 = Divide(x=w440, y=2) -> (x/y=w427:dbl)
                  n256 = Divide(x=w434, y=1000) -> (x/y=w444:sgl)
                  n257 = local read "Halt program"() -> (w439:bool)
                  n258 = Subtract(x=w427, y=w426) -> (x-y=w442:dbl)
                  n259 = Or(x=w439, y=w438) -> (x .or. y?=w435:bool)
                  n260 = Multiply(x=w444, y=w442) -> (x*y=w443:dbl)
                  n261 = Add(x=w430, y=w443) -> (x+y=w428:dbl)
                  n262 = invoke class="StepperMotorChannel" method="SetMoveAbsolutePosition"(reference=w432, error in=w431, "position"=w428) -> (reference out=w433:refnum<k24>, error out=w441:errorcluster)  [unwired: 1 in, 2 out]
                  n263 = invoke class="StepperMotorChannel" method="MoveAbsolute"(reference=w433, error in=w441, "waitTimeout"=20000) -> ()  [unwired: 1 in, 4 out]
                }
                frame #1 {
                  # "Inner loop: X-stepper"
                  n264 = while {
                    tunnel: w449 -> [w474]
                    tunnel: [w473] -> w456
                    tunnel: [w470] -> w458
                    tunnel: w452 -> [w463]
                    shift-right: [w468] -> w457
                    shift-left: w451 -> [w469]
                    tunnel: w450 -> [w467]
                    tunnel: [w466] -> w455
                    tunnel: [w465] -> w454
                    tunnel: w453 -> [w464]
                    tunnel: w448 -> [w462]
                    tunnel: w447 -> [w461]
                    tunnel: w446 -> [w460]
                    tunnel: [w459] -> w445
                    i -> [w472]
                    stop <- w471 stop-if-true
                    # "X-sequence: Move X, settle X, DAQ & plot"
                    n265 = stacked-sequence {
                      tunnel: w474 -> [_ _ w508]
                      tunnel: [w496 _ _] -> w473
                      tunnel: w464 -> [w495 _ _]
                      tunnel: w472 -> [w487 w499 w506]
                      tunnel: [w489 _ _] -> w471
                      tunnel: ["?" _ _] -> w470
                      tunnel: w469 -> [_ _ w513]
                      tunnel: [_ _ w511] -> w468
                      tunnel: w467 -> [_ _ w512]
                      tunnel: [_ _ w510] -> w466
                      tunnel: [_ _ w509] -> w465
                      tunnel: w463 -> [_ _ w505]
                      tunnel: w462 -> [w478 _ _]
                      tunnel: w461 -> [w477 _ _]
                      tunnel: w460 -> [_ _ w507]
                      tunnel: [w475 _ _] -> w459
                      frame #0 {
                        n266 = local read "Step Size X (um)"() -> (w479:sgl)
                        n267 = local read "Num Of Steps X"() -> (w485:i32)
                        n268 = Equal?(x=w487, y=w485) -> (x = y?=w492:bool)
                        n269 = Divide(x=w485, y=2) -> (x/y=w483:dbl)
                        n270 = Divide(x=w479, y=1000) -> (x/y=w480:sgl)
                        n271 = Subtract(x=w487, y=w483) -> (x-y=w486:dbl)
                        n272 = local read "Halt program"() -> (w491:bool)
                        n273 = Or(x=w491, y=w492) -> (x .or. y?=w490:bool)
                        n274 = Multiply(x=w480, y=w486) -> (x*y=w482:dbl)
                        n275 = Add(x=w477, y=w482) -> (x+y=w493:dbl)
                        n276 = invoke class="StepperMotorChannel" method="SetMoveAbsolutePosition"(reference=w478, error in=w495, "position"=w493) -> (reference out=w497:refnum<k24>, error out=w494:errorcluster)  [unwired: 1 in, 2 out]
                        n277 = invoke class="StepperMotorChannel" method="MoveAbsolute"(reference=w497, error in=w494, "waitTimeout"=0) -> (reference out=w496:refnum<k24>, error out=w475:errorcluster)  [unwired: 1 in, 2 out]
                        n278 = Or(x=w490, y="?") -> (x .or. y?=w489:bool)
                      }
                      frame #1 {
                        # "If i=0, it means we've likely just moved back to start of line, and we should wait a moment"
                        n279 = Equal?(x=0, y=w499) -> (x = y?=w500:bool)
                        n280 = case shown="True" w500 {
                          frame False {
                            n281 = Wait (ms)(milliseconds to wait="Settle Time X") -> ()  [unwired: 1 out]
                          }
                          frame True {
                            n282 = Wait (ms)(milliseconds to wait="Settle Time Y") -> ()  [unwired: 1 out]
                          }
                        }
                      }
                      frame #2 {
                        n283 = case shown="True" "Acquire" {
                          tunnel: w513 -> [w514 w544]
                          tunnel: w512 -> [w515 w540]
                          tunnel: [w514 w537] -> w511
                          tunnel: [w516 w533] -> w510
                          tunnel: [w515 w532] -> w509
                          tunnel: w508 -> [w516 w531]
                          tunnel: w507 -> [_ w530]
                          tunnel: w506 -> [_ w525]
                          tunnel: w505 -> [_ w524]
                          tunnel: "Integration time (s)" -> [w519 w522]
                          frame False {
                            n284 = Multiply(x=w519, y=1000) -> (x*y=w517:dbl)
                            n285 = Wait (ms)(milliseconds to wait=w517) -> ()  [unwired: 1 out]
                          }
                          frame True {
                            w552 = 200000
                            n286 = Multiply(x=w552, y=w522) -> (x*y=w551:dbl)
                            n287 = call "DAQ Assistant"("rate"=w552, "number of samples"=w551) -> ("data"=w550:dynamicdata)  [unwired: 15 in, 2 out]
                            n288 = call "Convert from Dynamic Data"("Dynamic Data Type"=w550) -> ("Array"=w549:dbl[][])  [unwired: 3 in]
                            n289 = Index Array(array=w549, index (row)=0) -> (element=w546:dbl[])  [unwired: 1 in]
                            n290 = Index Array(array=w549, index (row)=1) -> (element=w545:dbl[])  [unwired: 1 in]
                            n291 = call-poly <vilib>:"Mean.vi"("X"=w546) -> ("mean"=w541:dbl)  [unwired: 1 out]
                            n292 = call-poly <vilib>:"Mean.vi"("X"=w545) -> ("mean"=w529:dbl)  [unwired: 1 out]
                            n293 = Subtract(x=w541, y="1st sideband offset") -> (x-y=w523:dbl)
                            n294 = Multiply(x=w529, y="2nd sideband factor") -> (x*y=w528:dbl)
                            n295 = Re/Im To Complex(1:w528, 2:w523) -> (0:w526:cdb)
                            n296 = Replace Array Subset(array=w544, new element=w526, index (row)=w525, index (col)=w524) -> (w537:cdb[][])
                            n297 = Not(x="Auto-level phase") -> (.not. x?=w520:bool)
                            n298 = Complex To Polar(r * e^(i*theta)=w537) -> (r=→"Amplitude":dbl[][], theta=w539:dbl[][])
                            n299 = case shown="False" w520 {
                              tunnel: w540 -> [w574 w586]
                              tunnel: w539 -> [w573 w585]
                              tunnel: [w569 w584] -> w538
                              tunnel: "Phase offset" -> [w570 w583]
                              tunnel: "Px" -> [w572 w582]
                              tunnel: "Py" -> [w571 w581]
                              tunnel: [w567 w580] -> w533
                              tunnel: [w565 w579] -> w532
                              tunnel: w531 -> [w576 w578]
                              tunnel: w530 -> [w564 w577]
                              frame False {
                                n300 = node(w576, w564, "auto_phase_level", w574, w573, w573, w572, w571, w570) -> (w568:refnum<k35>, w566:errorcluster, w569:dbl[][])  [unwired: 4 in, 2 out]
                                n301 = Initialize Array(0.0, 3) -> (w553:dbl[])
                                n302 = node(w568, w564, "get_level_params", w566, w553, w553) -> (w567:refnum<k35>, w565:errorcluster, w559:dbl[])  [unwired: 1 in, 2 out]
                                n303 = Index Array(array=w559, index #1=0, index #2=1, index #3=2) -> (element #1=w562:dbl, element #2=w560:dbl, element #3=w561:dbl)
                                n304 = local write "Px"(w562) -> ()
                                n305 = local write "Py"(w560) -> ()
                                n306 = local write "Phase offset"(w561) -> ()
                              }
                              frame True {
                                n307 = node(w578, w577, "phase_level", w586, w585, w585, w582, w581, w583) -> (w580:refnum<k35>, w579:errorcluster, w584:dbl[][])  [unwired: 4 in, 2 out]
                              }
                            }
                            "Phase" <- w538
                          }
                        }
                      }
                    }
                  }
                }
              }
              n308 = Or(x=w425, y=w417) -> (x .or. y?=w424:bool)
            }
          }
          frame #2 {
            n309 = Wait (ms)(milliseconds to wait=1000) -> ()  [unwired: 1 out]
          }
          frame #3 {
            # "Return to origin postiion"
            n310 = invoke class="StepperMotorChannel" method="SetMoveAbsolutePosition"(reference=w590, "position"=w592) -> (reference out=w598:refnum<k24>, error out=w596:errorcluster)  [unwired: 2 in, 2 out]
            n311 = invoke class="StepperMotorChannel" method="MoveAbsolute"(reference=w598, error in=w596, "waitTimeout"=20000) -> ()  [unwired: 1 in, 4 out]
            n312 = invoke class="StepperMotorChannel" method="SetMoveAbsolutePosition"(reference=w589, "position"=w591) -> (reference out=w595:refnum<k24>, error out=w593:errorcluster)  [unwired: 2 in, 2 out]
            n313 = invoke class="StepperMotorChannel" method="MoveAbsolute"(reference=w595, error in=w593, "waitTimeout"=20000) -> ()  [unwired: 1 in, 4 out]
          }
          frame #4 {
            n314 = One Button Dialog(message="Scan Complete", button name ("OK")="OK") -> ()  [unwired: 1 out]
          }
        }
      }
    }
    n315 = local read "Halt program"() -> (w289:bool)
  }
  n316 = Close Python Session(session in=w21, error in=w20) -> ()  [unwired: 1 out]
  n317 = invoke class="StepperMotorChannel" method="Disconnect"(reference=w19, error in=w18) -> ()  [unwired: 1 in, 3 out]
